vi "Uploading dta file.vi"(8 "error in (no error)":errorcluster, 10 ".dta file Path":path=path "E:/VingCard/RFID_m645_Prodtest_LCU6331.128" caption="Path", 11 "VISA resource name":refnum<visa-resource-name>="COM2") -> (0 "error out":errorcluster, 2 "Pass?":bool, 3 "VISA resource name out":refnum<visa-resource-name>)   [LabVIEW 2009]
uses:
  <vilib>/Instr/_visa.llb/VISA Configure Serial Port (Instr).vi
panel:
  out "Uploading... .dta file":u8(slide) caption="Slide" scale=0.0..92.0
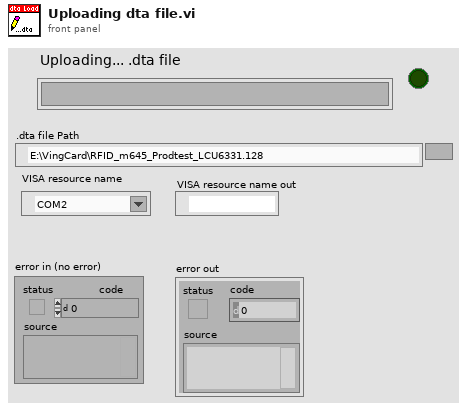
[diagram p1: front panel]
types:
  T1 = enum16{"change baud rate", "uploading dta file", "finish"}
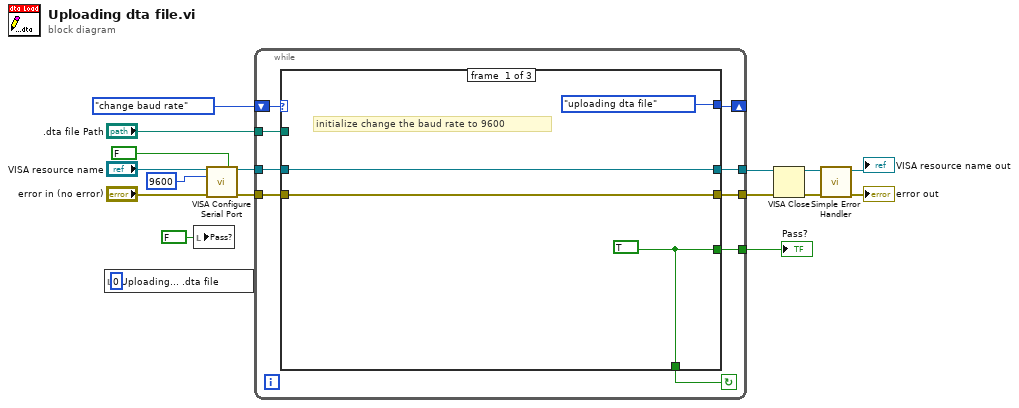
[diagram p0: block diagram]
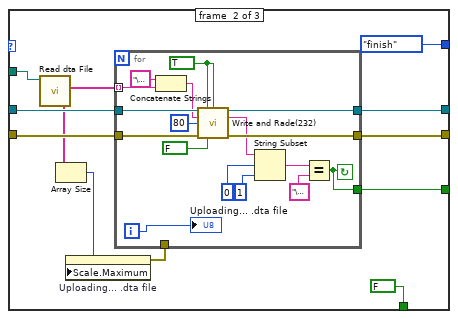
[diagram p2: hidden frame]
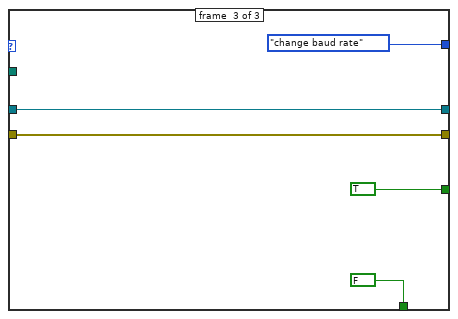
[diagram p3: hidden frame]
diagram:
  n1 = local write "Uploading... .dta file"(u8 0 ("Slide")) -> ()
  n2 = local write "Pass?"(FALSE ("Pass?")) -> ()
  n3 = call-poly "VISA Configure Serial Port"("VISA resource name"="VISA resource name", "Enable Termination\nChar (T)"=FALSE ("Enable Termination\nChar (T)"), "baud rate (9600)"=u32 9600, "error in (no error)"="error in (no error)") -> ("VISA resource name out"=w6:refnum<visa-resource-name>, "error out"=w5:errorcluster)  [unwired: 3 in, 7 out]
  n4 = while {
    shift-right: [w16] -> _
    shift-left: T1."change baud rate" -> [w24]
    tunnel: w6 -> [w22]
    tunnel: w5 -> [w21]
    tunnel: [w20] -> w13
    tunnel: [w19] -> w12
    tunnel: [w18] -> w11
    tunnel: ".dta file Path" -> [w17]
    stop <- w23 continue-if-true
    n5 = case shown="\"uploading dta file\"" w24 {
      tunnel: [T1."uploading dta file" T1."finish" T1."change baud rate"] -> w16
      tunnel: [w28 FALSE FALSE] -> w23
      tunnel: w22 -> [w26 w39 w60]
      tunnel: w21 -> [w25 w38 w59]
      tunnel: [w26 w37 w60] -> w20
      tunnel: [w25 w36 w59] -> w19
      tunnel: [w28 w35 TRUE] -> w18
      tunnel: w17 -> [_ w30 _]
      frame #0 {
        w28 = TRUE ("Enable Termination\nChar (T)")
        # "initialize change the baud rate to 9600"
      }
      frame #1 {
        n6 = call "Read dta File.vi"("Path"=w30) -> ("输出数组"=w33:string[])  [unwired: 1 in, 9 out]
        n7 = Array Size(array=w33) -> (size(s)=w32:i32)
        n8 = property on="Uploading... .dta file" class="Slide (strict)"("Scale.Maximum"=w32) -> (error out=w31:errorcluster)  [unwired: 2 in, 1 out]
        n9 = for {
          tunnel: w39 -> [w56]
          tunnel: w38 -> [w55]
          tunnel: [w54] -> w37
          tunnel: [w53] -> w36
          tunnel: w33 -> [w41] mode=indexing
          tunnel: [w45] -> w35
          tunnel: w31 -> [_]
          i -> [w44]
          stop <- w45 continue-if-true
          w47 = TRUE ("write")
          n10 = Concatenate Strings("\u0002" ("string"), w41) -> (w40:string)
          n11 = call "Write and Rade(232).vi"("VISA resource name in"=w56, "write"=w47, "read"=w47, "string to write"=w40, "ms delay"=u32 80 ("millisecond multiple"), "error in"=w55, "change baud rate(read)"=FALSE) -> ("VISA resource name out"=w54:refnum<visa-resource-name>, "read string"=w48:string, "error out"=w53:errorcluster)  [unwired: 1 in, 5 out]
          n12 = String Subset(string=w48, offset (0)=0, length (rest)=1 ("length (rest)")) -> (substring=w50:string)
          n13 = Equal?(x=w50, y="\u0006") -> (x = y?=w45:bool)
          "Uploading... .dta file" <- w44
        }
      }
      frame #2 {
      }
    }
  }
  "Pass?" <- w11
  "VISA resource name out" <- w13
  n14 = VISA Close(VISA resource name=w13, error in (no error)=w12) -> (error out=w14:errorcluster)
  n15 = call <vilib>:"Simple Error Handler.vi"("error in (no error)"=w14) -> ("error out"=→"error out":errorcluster)  [unwired: 1 in, 7 out]
